vi "getName.vi"(0 "Camera in":refnum<class "Camera.lvclass">, 11 "error in (no error)":errorcluster) -> (4 "Camera out":refnum<class "Camera.lvclass">, 6 "name":string, 15 "error out":errorcluster)   [LabVIEW 2019, in "Camera.lvclass"]
doc: "Retreive the rec handle.\nThis handle allows direct access to all underlying functions of the pco.recorder."
uses:
  Camera.lvclass
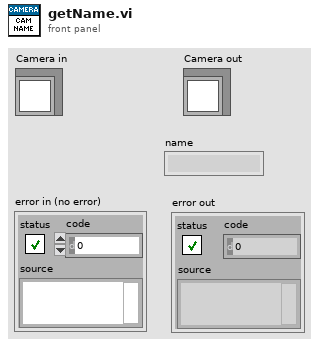
[diagram p1: front panel]
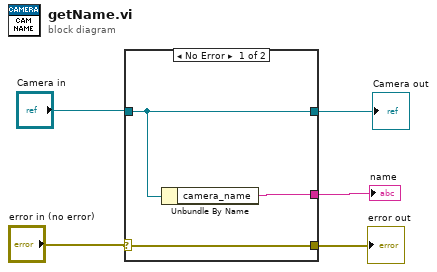
[diagram p0: block diagram]
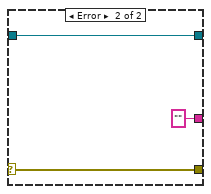
[diagram p2: hidden frame]
diagram:
  n1 = case shown="No Error" "error in (no error)" {
    selector: "error in (no error)" -> [w7 w11]
    tunnel: [w7 w11] -> w3
    tunnel: [w8 w10] -> w4
    tunnel: "Camera in" -> [w8 w10]
    tunnel: [w6 "" ("camera_name")] -> w1
    frame No Error {
      n2 = Unbundle By Name(w8) -> ("camera_name"=w6:string)
    }
    frame Error {
    }
  }
  "error out" <- w3
  "Camera out" <- w4
  "name" <- w1
